vi "Clawtest.vi"   [LabVIEW 2012]
uses:
  <vilib>/NXT/NXT Controls/ConnectionType.ctl
  <vilib>/NXT/Subs/MotorOutput.ctl
  <vilib>/NXT/Block Support/NXT_InputPort.ctl
types:
  T1 = typedef "ConnectionType.ctl" = enum16{"Bluetooth", "USB", "WiFi"}
  T2 = typedef "LVHSConnector.ctl" = refnum<class "BrickReference.lvclass">
  T3 = typedef "MotorOutput.ctl" = u8
  T4 = typedef "NXT_InputPort.ctl" = u8
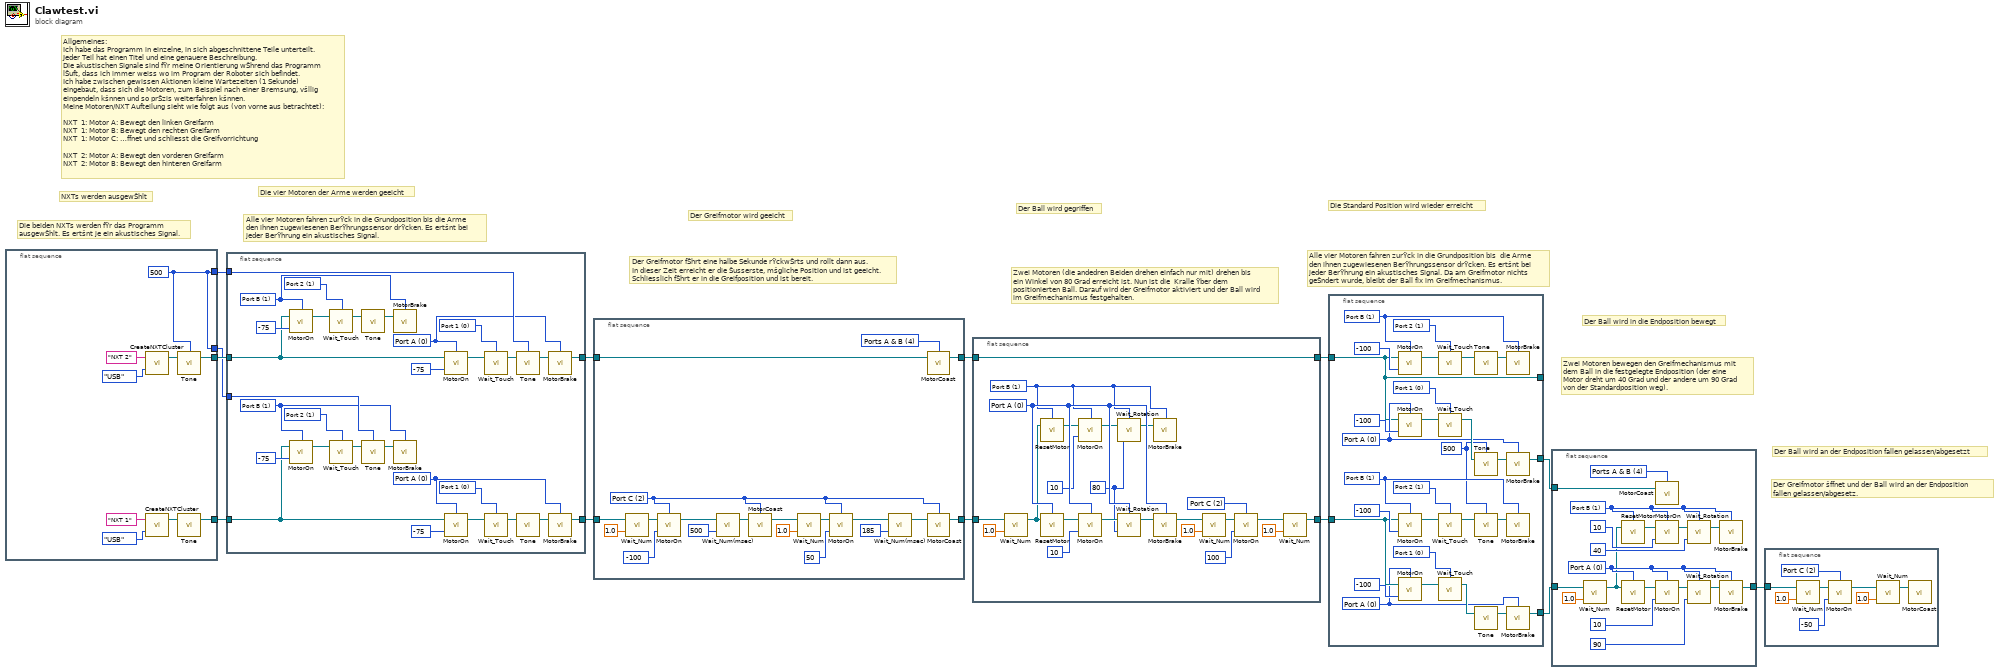
[diagram p0: block diagram]
diagram:
  # "Der Greifmotor šffnet und der Ball wird an der Endposition fallen gelassen/abgesetz."
  # "Der Ball wird an der Endposition fallen gelassen/abgesetzt"
  # "Zwei Motoren bewegen den Greifmechanismus mit\ndem Ball in die festgelegte Endposition (der eine \nMotor dreht um 40 Grad und der andere um 90 Grad \nvon der Standardposition weg)."
  # "Der Ball wird in die Endposition bewegt"
  # "Zwei Motoren (die andedren Beiden drehen einfach nur mit) drehen bis \nein Winkel von 80 Grad erreicht ist. Nun ist die  Kralle Ÿber dem\npositionierten Ball. Darauf wird der Greifmotor aktiviert und der Ball wird\nim Greifmechanismus festgehalten."
  # "Der Ball wird gegriffen"
  # "Alle vier Motoren fahren zurŸck in die Grundposition bis  die Arme\nden ihnen zugewiesenen BerŸhrungssensor drŸcken. Es ertšnt bei \njeder BerŸhrung ein akustisches Signal. Da am Greifmotor nichts \ngeŠndert wurde, bleibt der Ball fix im Greifmechanismus."
  # "Die Standard Position wird wieder erreicht"
  # "Allgemeines:\nIch habe das Programm in einzelne, in sich abgeschnittene Teile unterteilt. \nJeder Teil hat einen Titel und eine genauere Beschreibung.\nDie akustischen Signale sind fŸr meine Orientierung wŠhrend das Programm \nlŠuft, dass ich immer weiss wo im Program der Roboter sich befindet.\nIch habe zwischen gewissen Aktionen kleine Wartezeiten (1 Sekunde)\neingebaut, dass sich die Motoren, zum Beispiel nach einer Bremsung, všllig\neinpendeln kšnnen und so prŠzis weiterfahren kšnnen.\nMeine Motoren/NXT Aufteilung sieht wie folgt aus (von vorne aus betrachtet):\n\nNXT  1: Motor A: Bewegt den linken Greifarm \nNXT  1: Motor B: Bewegt den rechten Greifarm\nNXT  1: Motor C: …ffnet und schliesst die Greifvorrichtung \n\nNXT  2: Motor A: Bewegt den vorderen Greifarm\nNXT  2: Motor B: Bewegt den hinteren Greifarm"
  # "Der Greifmotor fŠhrt eine halbe Sekunde rŸckwŠrts und rollt dann aus. \nIn dieser Zeit erreicht er die Šusserste, mšgliche Position und ist geeicht.\nSchliesslich fŠhrt er in die Greifposition und ist bereit."
  # "Der Greifmotor wird geeicht"
  # "Die vier Motoren der Arme werden geeicht"
  # "NXTs werden ausgewŠhlt"
  # "Alle vier Motoren fahren zurŸck in die Grundposition bis die Arme\nden ihnen zugewiesenen BerŸhrungssensor drŸcken. Es ertšnt bei \njeder BerŸhrung ein akustisches Signal."
  # "Die beiden NXTs werden fŸr das Programm \nausgewŠhlt. Es ertšnt je ein akustisches Signal."
  n1 = flat-sequence {
    tunnel: [w17] -> w13
    tunnel: [w15] -> w12
    tunnel: [w14] -> w11
    tunnel: [w14] -> w10
    frame #0 {
      w14 = u16 500 ("Tone (440 Hz)")
      n2 = call <vilib>:"CreateNXTCluster.vi"("Connection Type"=ConnectionType."USB", "NXT name"="NXT 2") -> ("NXT"=w16:T2)  [unwired: 2 in]
      n3 = call <vilib>:"CreateNXTCluster.vi"("Connection Type"=ConnectionType."USB", "NXT name"="NXT 1") -> ("NXT"=w18:T2)  [unwired: 2 in]
      n4 = call <vilib>:"Tone.vi"("NXT"=w16, "Tone (440 Hz)"=w14) -> ("NXT"=w15:T2)  [unwired: 2 in]
      n5 = call <vilib>:"Tone.vi"("NXT"=w18) -> ("NXT"=w17:T2)  [unwired: 3 in]
    }
  }
  n6 = flat-sequence {
    tunnel: w13 -> [w44]
    tunnel: w12 -> [w43]
    tunnel: w11 -> [w31]
    tunnel: w10 -> [w30]
    tunnel: [w29] -> w9
    tunnel: [w24] -> w8
    frame #0 {
      w27 = T3 1 items=["Port A"=0, "Port B"=1, "Port C"=2, "Ports A & B"=4, "Ports A & C"=5, "Ports B & C"=6, "All Ports"=3] ("Output Port (All Ports)")
      w39 = T4 1 items=["Port 1", "Port 2", "Port 3", "Port 4"] ("Port (Port 1)")
      w38 = T4 0 items=["Port 1", "Port 2", "Port 3", "Port 4"] ("Port (Port 1)")
      w28 = T3 1 items=["Port A"=0, "Port B"=1, "Port C"=2, "Ports A & B"=4, "Ports A & C"=5, "Ports B & C"=6, "All Ports"=3] ("Output Port (All Ports)")
      w23 = T3 0 items=["Port A"=0, "Port B"=1, "Port C"=2, "Ports A & B"=4, "Ports A & C"=5, "Ports B & C"=6, "All Ports"=3] ("Output Port (All Ports)")
      w40 = T4 1 items=["Port 1", "Port 2", "Port 3", "Port 4"] ("Port (Port 1)")
      w26 = T4 0 items=["Port 1", "Port 2", "Port 3", "Port 4"] ("Port (Port 1)")
      w25 = T3 0 items=["Port A"=0, "Port B"=1, "Port C"=2, "Ports A & B"=4, "Ports A & C"=5, "Ports B & C"=6, "All Ports"=3] ("Output Port (All Ports)")
      n7 = call <vilib>:"MotorOn.vi"("Power (75)"=-75, "NXT"=w43, "Output Port (All Ports)"=w28) -> ("NXT"=w45:T2)  [unwired: 1 in]
      n8 = call <vilib>:"MotorOn.vi"("Power (75)"=-75, "NXT"=w44, "Output Port (All Ports)"=w27) -> ("NXT"=w49:T2)  [unwired: 1 in]
      n9 = call <vilib>:"Wait_Touch.vi"("NXT"=w45, "Port (Port 1)"=w39) -> ("NXT"=w35:T2)  [unwired: 2 in]
      n10 = call <vilib>:"Wait_Touch.vi"("NXT"=w49, "Port (Port 1)"=w40) -> ("NXT"=w37:T2)  [unwired: 2 in]
      n11 = call <vilib>:"Tone.vi"("NXT"=w35) -> ("NXT"=w34:T2)  [unwired: 3 in]
      n12 = call <vilib>:"Tone.vi"("NXT"=w37, "Tone (440 Hz)"=w31) -> ("NXT"=w36:T2)  [unwired: 2 in]
      n13 = call <vilib>:"MotorBrake.vi"("NXT"=w34, "Port (All Ports)"=w28) -> ()  [unwired: 2 in, 1 out]
      n14 = call <vilib>:"MotorBrake.vi"("NXT"=w36, "Port (All Ports)"=w27) -> ()  [unwired: 2 in, 1 out]
      n15 = call <vilib>:"MotorOn.vi"("Power (75)"=-75, "NXT"=w43, "Output Port (All Ports)"=w23) -> ("NXT"=w46:T2)  [unwired: 1 in]
      n16 = call <vilib>:"MotorOn.vi"("Power (75)"=-75, "NXT"=w44, "Output Port (All Ports)"=w25) -> ("NXT"=w50:T2)  [unwired: 1 in]
      n17 = call <vilib>:"Wait_Touch.vi"("NXT"=w46, "Port (Port 1)"=w38) -> ("NXT"=w33:T2)  [unwired: 2 in]
      n18 = call <vilib>:"Wait_Touch.vi"("NXT"=w50, "Port (Port 1)"=w26) -> ("NXT"=w42:T2)  [unwired: 2 in]
      n19 = call <vilib>:"Tone.vi"("NXT"=w33, "Tone (440 Hz)"=w30) -> ("NXT"=w32:T2)  [unwired: 2 in]
      n20 = call <vilib>:"Tone.vi"("NXT"=w42) -> ("NXT"=w41:T2)  [unwired: 3 in]
      n21 = call <vilib>:"MotorBrake.vi"("NXT"=w32, "Port (All Ports)"=w23) -> ("NXT"=w29:T2)  [unwired: 2 in]
      n22 = call <vilib>:"MotorBrake.vi"("NXT"=w41, "Port (All Ports)"=w25) -> ("NXT"=w24:T2)  [unwired: 2 in]
    }
  }
  n23 = flat-sequence {
    tunnel: w9 -> [w58]
    tunnel: w8 -> [w56]
    tunnel: [w54] -> w4
    tunnel: [w53] -> w2
    frame #0 {
      w70 = T3 2 items=["Port A"=0, "Port B"=1, "Port C"=2, "Ports A & B"=4, "Ports A & C"=5, "Ports B & C"=6, "All Ports"=3] ("Output Port (All Ports)")
      w71 = T3 4 items=["Port A"=0, "Port B"=1, "Port C"=2, "Ports A & B"=4, "Ports A & C"=5, "Ports B & C"=6, "All Ports"=3] ("Port (All Ports)")
      n24 = call <vilib>:"Wait_Num.vi"("Time (1 sec)"=sgl 1.0, "NXT"=w56) -> ("NXT"=w55:T2)  [unwired: 2 in]
      n25 = call <vilib>:"MotorOn.vi"("Power (75)"=-100, "NXT"=w55, "Output Port (All Ports)"=w70) -> ("NXT"=w59:T2)  [unwired: 1 in]
      n26 = call <vilib>:"Wait_Num(msec).vi"("Time (100 msec)"=u32 500, "NXT"=w59) -> ("NXT"=w60:T2)  [unwired: 2 in]
      n27 = call <vilib>:"MotorCoast.vi"("NXT"=w60, "Port (All Ports)"=w70) -> ("NXT"=w69:T2)  [unwired: 2 in]
      n28 = call <vilib>:"Wait_Num.vi"("Time (1 sec)"=sgl 1.0, "NXT"=w69) -> ("NXT"=w68:T2)  [unwired: 2 in]
      n29 = call <vilib>:"MotorOn.vi"("Power (75)"=50, "NXT"=w68, "Output Port (All Ports)"=w70) -> ("NXT"=w63:T2)  [unwired: 1 in]
      n30 = call <vilib>:"Wait_Num(msec).vi"("Time (100 msec)"=u32 185, "NXT"=w63) -> ("NXT"=w64:T2)  [unwired: 2 in]
      n31 = call <vilib>:"MotorCoast.vi"("NXT"=w58, "Port (All Ports)"=w71) -> ("NXT"=w53:T2)  [unwired: 2 in]
      n32 = call <vilib>:"MotorCoast.vi"("NXT"=w64, "Port (All Ports)"=w70) -> ("NXT"=w54:T2)  [unwired: 2 in]
    }
  }
  n33 = flat-sequence {
    tunnel: [w76] -> w5
    tunnel: w4 -> [w74]
    tunnel: [w73] -> w3
    tunnel: w2 -> [w73]
    frame #0 {
      w72 = 80 ("Position Change (180)")
      w92 = T3 2 items=["Port A"=0, "Port B"=1, "Port C"=2, "Ports A & B"=4, "Ports A & C"=5, "Ports B & C"=6, "All Ports"=3] ("Output Port (All Ports)")
      w87 = T3 1 items=["Port A"=0, "Port B"=1, "Port C"=2, "Ports A & B"=4, "Ports A & C"=5, "Ports B & C"=6, "All Ports"=3] ("Port (All Ports)")
      w88 = T3 0 items=["Port A"=0, "Port B"=1, "Port C"=2, "Ports A & B"=4, "Ports A & C"=5, "Ports B & C"=6, "All Ports"=3] ("Port (All Ports)")
      n34 = call <vilib>:"Wait_Num.vi"("Time (1 sec)"=sgl 1.0, "NXT"=w74) -> ("NXT"=w75:T2)  [unwired: 2 in]
      n35 = call <vilib>:"ResetMotor.vi"("NXT"=w75, "Port (All Ports)"=w87) -> ("NXT"=w85:T2)  [unwired: 2 in]
      n36 = call <vilib>:"ResetMotor.vi"("NXT"=w75, "Port (All Ports)"=w88) -> ("NXT"=w77:T2)  [unwired: 2 in]
      n37 = call <vilib>:"MotorOn.vi"("Power (75)"=10, "NXT"=w85, "Output Port (All Ports)"=w87) -> ("NXT"=w86:T2)  [unwired: 1 in]
      n38 = call <vilib>:"MotorOn.vi"("Power (75)"=10, "NXT"=w77, "Output Port (All Ports)"=w88) -> ("NXT"=w78:T2)  [unwired: 1 in]
      n39 = call <vilib>:"Wait_Rotation.vi"("Position Change (180)"=w72, "NXT"=w86, "Port (Port A)"=w87) -> ("NXT"=w83:T2)  [unwired: 1 in]
      n40 = call <vilib>:"Wait_Rotation.vi"("Position Change (180)"=w72, "NXT"=w78, "Port (Port A)"=w88) -> ("NXT"=w80:T2)  [unwired: 1 in]
      n41 = call <vilib>:"MotorBrake.vi"("NXT"=w83, "Port (All Ports)"=w87) -> ()  [unwired: 2 in, 1 out]
      n42 = call <vilib>:"MotorBrake.vi"("NXT"=w80, "Port (All Ports)"=w88) -> ("NXT"=w81:T2)  [unwired: 2 in]
      n43 = call <vilib>:"Wait_Num.vi"("Time (1 sec)"=sgl 1.0, "NXT"=w81) -> ("NXT"=w91:T2)  [unwired: 2 in]
      n44 = call <vilib>:"MotorOn.vi"("Power (75)"=100, "NXT"=w91, "Output Port (All Ports)"=w92) -> ("NXT"=w94:T2)  [unwired: 1 in]
      n45 = call <vilib>:"Wait_Num.vi"("Time (1 sec)"=sgl 1.0, "NXT"=w94) -> ("NXT"=w76:T2)  [unwired: 2 in]
    }
  }
  n46 = flat-sequence {
    tunnel: w5 -> [w115]
    tunnel: [w96] -> _
    tunnel: [w103] -> w7
    tunnel: [w97] -> w6
    tunnel: w3 -> [w96]
    frame #0 {
      w95 = u16 500 ("Tone (440 Hz)")
      w100 = T3 1 items=["Port A"=0, "Port B"=1, "Port C"=2, "Ports A & B"=4, "Ports A & C"=5, "Ports B & C"=6, "All Ports"=3] ("Output Port (All Ports)")
      w111 = T4 1 items=["Port 1", "Port 2", "Port 3", "Port 4"] ("Port (Port 1)")
      w110 = T4 0 items=["Port 1", "Port 2", "Port 3", "Port 4"] ("Port (Port 1)")
      w102 = T3 1 items=["Port A"=0, "Port B"=1, "Port C"=2, "Ports A & B"=4, "Ports A & C"=5, "Ports B & C"=6, "All Ports"=3] ("Output Port (All Ports)")
      w101 = T3 0 items=["Port A"=0, "Port B"=1, "Port C"=2, "Ports A & B"=4, "Ports A & C"=5, "Ports B & C"=6, "All Ports"=3] ("Output Port (All Ports)")
      w112 = T4 1 items=["Port 1", "Port 2", "Port 3", "Port 4"] ("Port (Port 1)")
      w99 = T4 0 items=["Port 1", "Port 2", "Port 3", "Port 4"] ("Port (Port 1)")
      w98 = T3 0 items=["Port A"=0, "Port B"=1, "Port C"=2, "Ports A & B"=4, "Ports A & C"=5, "Ports B & C"=6, "All Ports"=3] ("Output Port (All Ports)")
      n47 = call <vilib>:"MotorOn.vi"("Power (75)"=-100, "NXT"=w96, "Output Port (All Ports)"=w102) -> ("NXT"=w116:T2)  [unwired: 1 in]
      n48 = call <vilib>:"MotorOn.vi"("Power (75)"=-100, "NXT"=w96, "Output Port (All Ports)"=w101) -> ("NXT"=w117:T2)  [unwired: 1 in]
      n49 = call <vilib>:"MotorOn.vi"("Power (75)"=-100, "NXT"=w115, "Output Port (All Ports)"=w100) -> ("NXT"=w120:T2)  [unwired: 1 in]
      n50 = call <vilib>:"MotorOn.vi"("Power (75)"=-100, "NXT"=w115, "Output Port (All Ports)"=w98) -> ("NXT"=w121:T2)  [unwired: 1 in]
      n51 = call <vilib>:"Wait_Touch.vi"("NXT"=w116, "Port (Port 1)"=w111) -> ("NXT"=w107:T2)  [unwired: 2 in]
      n52 = call <vilib>:"Wait_Touch.vi"("NXT"=w117, "Port (Port 1)"=w110) -> ("NXT"=w105:T2)  [unwired: 2 in]
      n53 = call <vilib>:"Wait_Touch.vi"("NXT"=w120, "Port (Port 1)"=w112) -> ("NXT"=w109:T2)  [unwired: 2 in]
      n54 = call <vilib>:"Wait_Touch.vi"("NXT"=w121, "Port (Port 1)"=w99) -> ("NXT"=w114:T2)  [unwired: 2 in]
      n55 = call <vilib>:"Tone.vi"("NXT"=w107) -> ("NXT"=w106:T2)  [unwired: 3 in]
      n56 = call <vilib>:"Tone.vi"("NXT"=w105, "Tone (440 Hz)"=w95) -> ("NXT"=w104:T2)  [unwired: 2 in]
      n57 = call <vilib>:"Tone.vi"("NXT"=w109, "Tone (440 Hz)"=w95) -> ("NXT"=w108:T2)  [unwired: 2 in]
      n58 = call <vilib>:"Tone.vi"("NXT"=w114) -> ("NXT"=w113:T2)  [unwired: 3 in]
      n59 = call <vilib>:"MotorBrake.vi"("NXT"=w106, "Port (All Ports)"=w102) -> ()  [unwired: 2 in, 1 out]
      n60 = call <vilib>:"MotorBrake.vi"("NXT"=w104, "Port (All Ports)"=w101) -> ("NXT"=w103:T2)  [unwired: 2 in]
      n61 = call <vilib>:"MotorBrake.vi"("NXT"=w108, "Port (All Ports)"=w100) -> ()  [unwired: 2 in, 1 out]
      n62 = call <vilib>:"MotorBrake.vi"("NXT"=w113, "Port (All Ports)"=w98) -> ("NXT"=w97:T2)  [unwired: 2 in]
    }
  }
  n63 = flat-sequence {
    tunnel: w7 -> [w128]
    tunnel: w6 -> [w126]
    tunnel: [w124] -> w1
    frame #0 {
      w129 = T3 4 items=["Port A"=0, "Port B"=1, "Port C"=2, "Ports A & B"=4, "Ports A & C"=5, "Ports B & C"=6, "All Ports"=3] ("Port (All Ports)")
      w133 = T3 1 items=["Port A"=0, "Port B"=1, "Port C"=2, "Ports A & B"=4, "Ports A & C"=5, "Ports B & C"=6, "All Ports"=3] ("Port (All Ports)")
      w132 = T3 0 items=["Port A"=0, "Port B"=1, "Port C"=2, "Ports A & B"=4, "Ports A & C"=5, "Ports B & C"=6, "All Ports"=3] ("Port (All Ports)")
      n64 = call <vilib>:"Wait_Num.vi"("Time (1 sec)"=sgl 1.0, "NXT"=w126) -> ("NXT"=w125:T2)  [unwired: 2 in]
      n65 = call <vilib>:"ResetMotor.vi"("NXT"=w125, "Port (All Ports)"=w133) -> ("NXT"=w135:T2)  [unwired: 2 in]
      n66 = call <vilib>:"ResetMotor.vi"("NXT"=w125, "Port (All Ports)"=w132) -> ("NXT"=w141:T2)  [unwired: 2 in]
      n67 = call <vilib>:"MotorCoast.vi"("NXT"=w128, "Port (All Ports)"=w129) -> ()  [unwired: 2 in, 1 out]
      n68 = call <vilib>:"MotorOn.vi"("Power (75)"=10, "NXT"=w135, "Output Port (All Ports)"=w133) -> ("NXT"=w134:T2)  [unwired: 1 in]
      n69 = call <vilib>:"MotorOn.vi"("Power (75)"=10, "NXT"=w141, "Output Port (All Ports)"=w132) -> ("NXT"=w140:T2)  [unwired: 1 in]
      n70 = call <vilib>:"Wait_Rotation.vi"("Position Change (180)"=40, "NXT"=w134, "Port (Port A)"=w133) -> ("NXT"=w137:T2)  [unwired: 1 in]
      n71 = call <vilib>:"Wait_Rotation.vi"("Position Change (180)"=90, "NXT"=w140, "Port (Port A)"=w132) -> ("NXT"=w138:T2)  [unwired: 1 in]
      n72 = call <vilib>:"MotorBrake.vi"("NXT"=w137, "Port (All Ports)"=w133) -> ()  [unwired: 2 in, 1 out]
      n73 = call <vilib>:"MotorBrake.vi"("NXT"=w138, "Port (All Ports)"=w132) -> ("NXT"=w124:T2)  [unwired: 2 in]
    }
  }
  n74 = flat-sequence {
    tunnel: w1 -> [w143]
    frame #0 {
      w149 = T3 2 items=["Port A"=0, "Port B"=1, "Port C"=2, "Ports A & B"=4, "Ports A & C"=5, "Ports B & C"=6, "All Ports"=3] ("Output Port (All Ports)")
      n75 = call <vilib>:"Wait_Num.vi"("Time (1 sec)"=sgl 1.0, "NXT"=w143) -> ("NXT"=w144:T2)  [unwired: 2 in]
      n76 = call <vilib>:"MotorOn.vi"("Power (75)"=-50, "NXT"=w144, "Output Port (All Ports)"=w149) -> ("NXT"=w146:T2)  [unwired: 1 in]
      n77 = call <vilib>:"Wait_Num.vi"("Time (1 sec)"=sgl 1.0, "NXT"=w146) -> ("NXT"=w145:T2)  [unwired: 2 in]
      n78 = call <vilib>:"MotorCoast.vi"("NXT"=w145) -> ()  [unwired: 3 in, 1 out]
    }
  }
